vi "BuildDeltaString.vi"(1 "L*a*b":dbl[][](array[numeric])) -> (0 "DeltaEString":string[](array[string]))   [LabVIEW 2013]
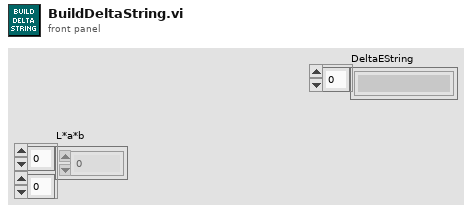
[diagram p1: front panel]
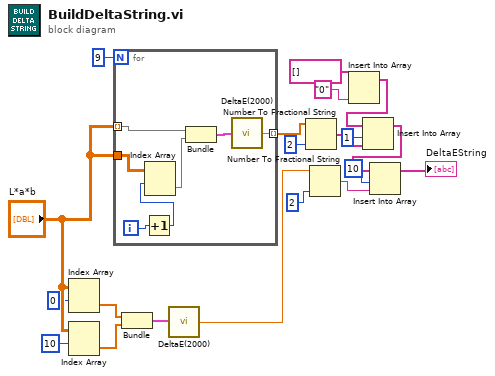
[diagram p0: block diagram]
diagram:
  n1 = Index Array(array="L*a*b", index (row)=0) -> (element=w14:dbl[])  [unwired: 1 in]
  n2 = Index Array(array="L*a*b", index (row)=10) -> (element=w13:dbl[])  [unwired: 1 in]
  n3 = for {
    N: 9 -> [_]
    tunnel: "L*a*b" -> [w26] mode=indexing
    tunnel: "L*a*b" -> [w25]
    tunnel: [w21] -> w19 mode=indexing
    i -> [w27]
    n4 = Increment(x=w27) -> (x+1=w24:i32)
    n5 = Index Array(array=w25, index (row)=w24) -> (element=w23:dbl[])  [unwired: 1 in]
    n6 = Bundle("L*a*b"=w26, "L*a*b"=w23) -> (w22:cluster{"L*a*b":dbl[], "L*a*b":dbl[]})  [unwired: 1 in]
    n7 = call "DeltaE(2000).vi"("L*a*b Colors"=w22) -> ("Delta E"=w21:dbl)
  }
  n8 = Bundle("L*a*b"=w14, "L*a*b"=w13) -> (w12:cluster{"L*a*b":dbl[], "L*a*b":dbl[]})  [unwired: 1 in]
  n9 = call "DeltaE(2000).vi"("L*a*b Colors"=w12) -> ("Delta E"=w10:dbl)
  n10 = Number To Fractional String(number=w19, precision (6)=i16 2) -> (F-format string=w7:string[])  [unwired: 2 in]
  n11 = Number To Fractional String(number=w10, precision (6)=i16 2) -> (F-format string=w2:string)  [unwired: 2 in]
  n12 = Insert Into Array(array=string[] [], new element="0") -> (w6:string[])  [unwired: 1 in]
  n13 = Insert Into Array(array=w6, index=1, new element=w7) -> (w4:string[])
  n14 = Insert Into Array(array=w4, index=10, new element=w2) -> (→"DeltaEString":string[])
